vi "FINAL.vi"() -> ()   [LabVIEW 2018]
uses:
  <vilib>/Tufts CEEO ROS for LabVIEW Software/ROS/Code/SubVIs/_ROSControl.ctl
  <vilib>/Tufts CEEO ROS for LabVIEW Software/ROS/Code/SubVIs/_ROSDirection.ctl
  <vilib>/Tufts CEEO ROS for LabVIEW Software/ROS/Code/Console/Servers/ServerSubs/TopicDef.ctl
  <vilib>/Tufts CEEO ROS for LabVIEW Software/ROS/MessageBuilding/std_msgs/subs/stringScalar.vi
panel:
  in  "START/STOP":bool
  out "Robot state":bool
  in  "Manual/AUTONOMOUS":bool
  in  "LEFT":bool
  in  "DOWN":bool
  in  "RIGHT":bool
  in  "TOP":bool
  in  "Y POSITION":dbl
  in  "THETA POSITION":dbl
  in  "X POSITION":dbl
  out "ROBOT SPEED":dbl(knob) scale=0.0..10.0
  out "ROS out":T1={"topic port"=0, "Node"="", "topic"="", "type"="", "node port"=0, "error "={"status"=FALSE, "code"=0, "source"=""}, "Direction"=enum."Node", "Update (ms)"=1, "FIFO size"=1}
  out "error out":errorcluster
  out "position graph":cluster{"X":dbl, "Y":dbl}[](graph)
  out "obstacles graph":cluster{"X":dbl, "Y":dbl}[](graph)
  # "Robot state"
  # "MANUAL MODE"
  # "CONTROL\nMODE"
  # "AUTONOMOUS MODE"
  # "MANUAL MODE"
  # "AUTONOMOUS MODE"
  # "ROBOT SPEED"
  # "ROBOT POSITION IN THE MAP"
  # "LASER SCAN PLOT"
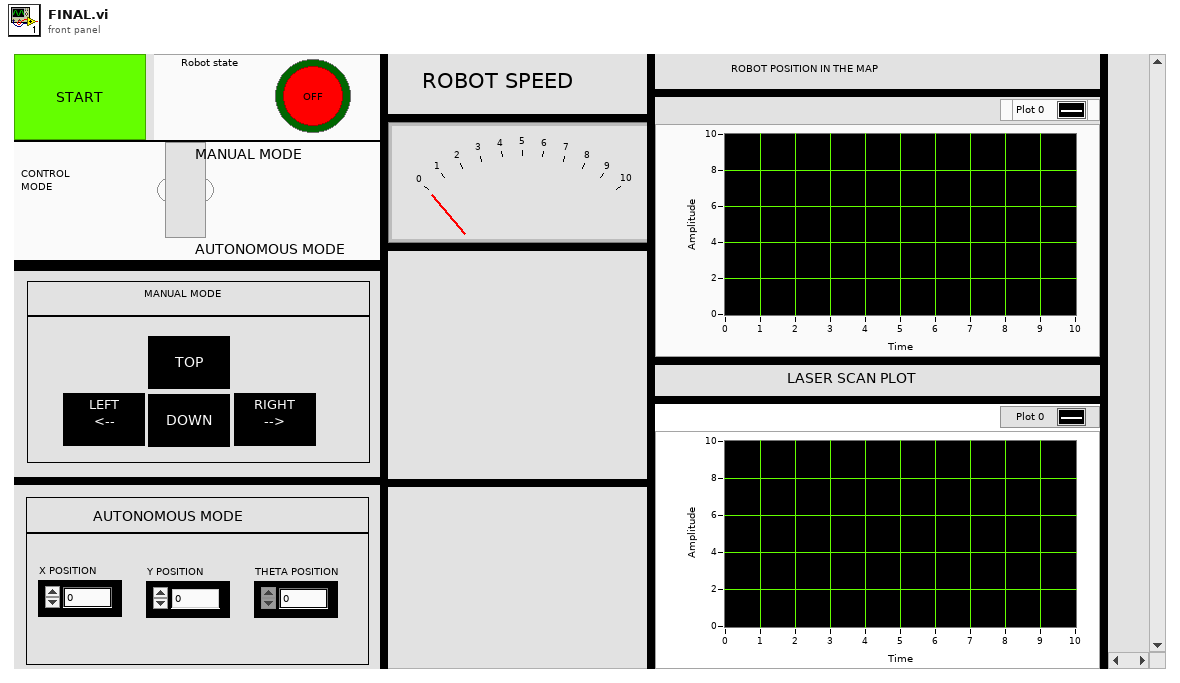
[diagram p1: front panel]
types:
  T1 = typedef "_ROSControl.ctl" = cluster{"topic port":u16, "Node":string, "topic":string, "type":string, "node port":u16, "error ":errorcluster, "Direction":T2, "Update (ms)":u16, "FIFO size":u16}
  T2 = typedef "_ROSDirection.ctl" = enum16{"Node", "Publisher", "Subscriber", "ServiceClient", "ServiceProvider"}
  T3 = typedef "TopicDef.ctl" = cluster{"Topic":string, "Type":string, "Action":T2, "Update (ms)":u16, "queue size":u16}
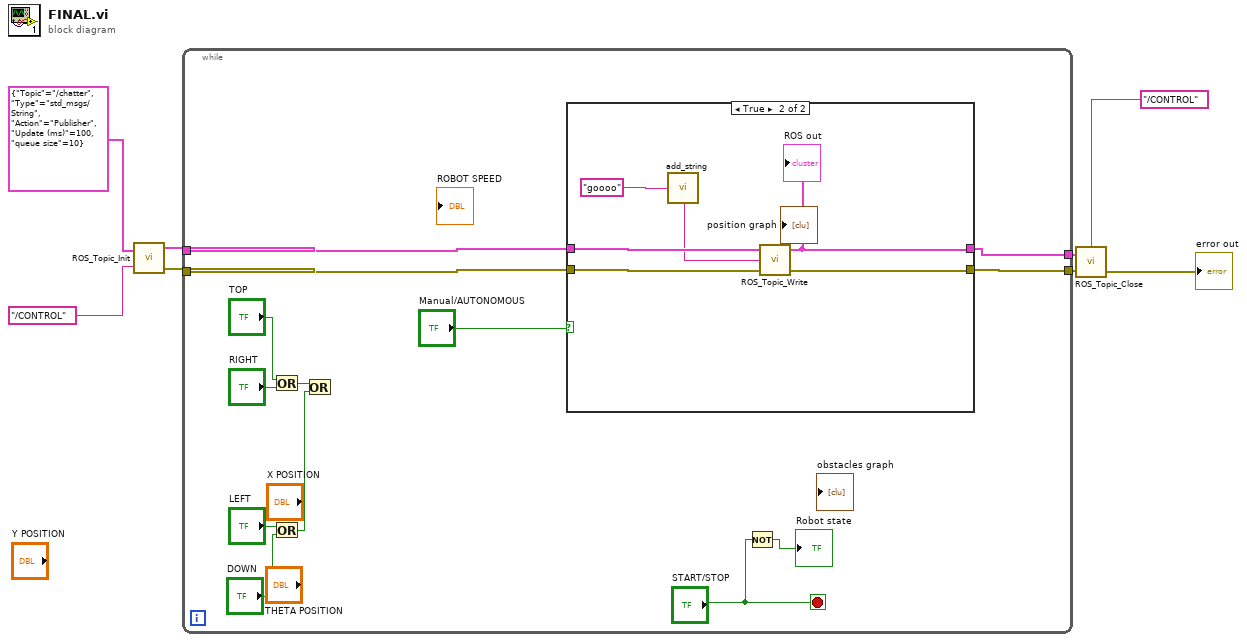
[diagram p0: block diagram]
diagram:
  n1 = call <vilib>:"ROS_Topic_Init.vi"("Definitions"=T3 {"Topic"="/chatter", "Type"="std_msgs/String", "Action"=enum."Publisher", "Update (ms)"=100, "queue size"=10}, "node"="/CONTROL") -> ("ROS out"=w7:T1, "error out"=w8:errorcluster)  [unwired: 1 in]
  n2 = while {
    tunnel: w8 -> [w15]
    tunnel: w7 -> [w14]
    tunnel: [w10] -> w2
    tunnel: [w9] -> w1
    stop <- "START/STOP" stop-if-true
    n3 = Or(x="TOP", y="RIGHT") -> (x .or. y?=w17:bool)
    n4 = Or(x="LEFT", y="DOWN") -> (x .or. y?=w16:bool)
    n5 = Or(x=w17, y=w16) -> ()  [unwired: 1 out]
    n6 = case shown="True" "Manual/AUTONOMOUS" {
      tunnel: w15 -> [w22 w29]
      tunnel: w14 -> [w23 w28]
      tunnel: [w23 w25] -> w10
      tunnel: [w22 w27] -> w9
      frame False {
      }
      frame True {
        n7 = call-poly <vilib>:"add_string.vi"("String"="goooo") -> ("msg out"=w26:string)  [unwired: 4 in]
        n8 = call <vilib>:"ROS_Topic_Write.vi"("error in (no error)"=w29, "Msg in"=w26, "ROS in"=w28) -> ("error out"=w27:errorcluster, "ROS out"=w25:T1)  [unwired: 1 in]
        "ROS out" <- w25
      }
    }
    n9 = Not(x="START/STOP") -> (.not. x?=→"Robot state":bool)
  }
  n10 = call <vilib>:"ROS_Topic_Close.vi"("error in"=w1, "ROS in"=w2, "node"="/CONTROL") -> ("error out"=→"error out":errorcluster)  [unwired: 1 in]
